vi "Plot 4 corners.vi"(8 "error in (no error)":errorcluster, 10 "4 corners":dbl[][][](array[numeric]), 11 "Refnum in":T1) -> (0 "error out":errorcluster, 3 "Refnum out":T1)   [LabVIEW 2011]
uses:
  <vilib>/vision/Image Controls.llb/IMAQ Image.ctl
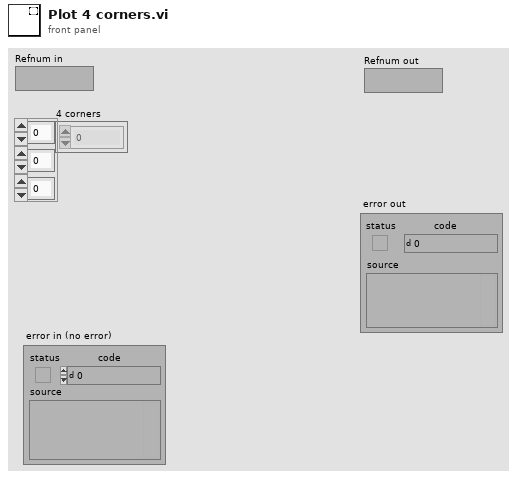
[diagram p1: front panel]
types:
  T1 = typedef "IMAQ Image.ctl" = refnum<image>
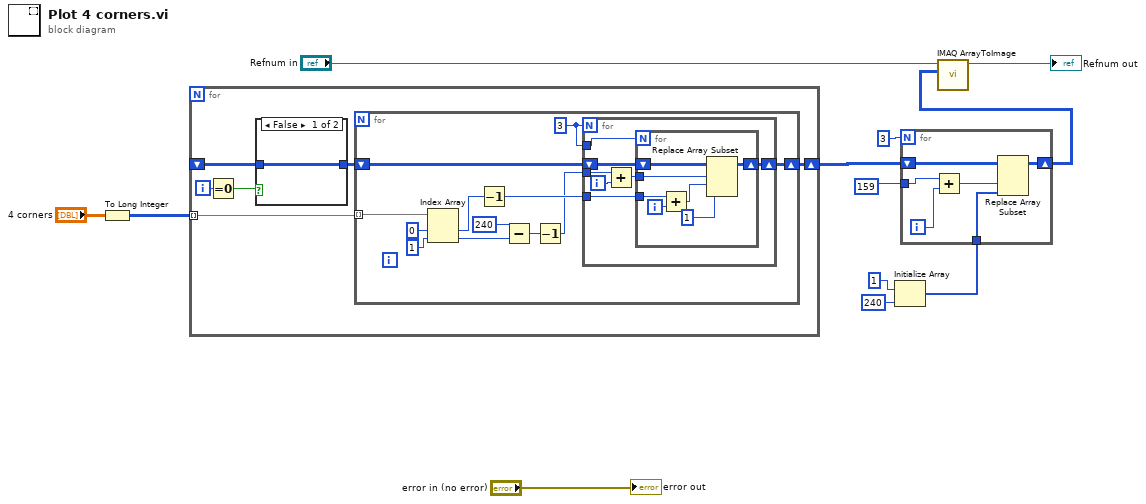
[diagram p0: block diagram]
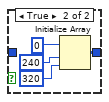
[diagram p2: hidden frame]
diagram:
  n1 = To Long Integer(number="4 corners") -> (32bit integer=w8:i32[][][])
  n2 = for {
    tunnel: w8 -> [w17] mode=indexing
    shift-right: [w16] -> w7
    shift-left: _ -> [w13]
    i -> [w15]
    n3 = Equal To 0?(x=w15) -> (x = 0?=w14:bool)
    n4 = case shown="False" w14 {
      tunnel: [w19 w20] -> w18
      tunnel: w13 -> [w19 _]
      frame False {
      }
      frame True {
        n5 = Initialize Array(u8 0, 240 ("dimension size"), 320 ("dimension size")) -> (w20:u8[][])
      }
    }
    n6 = for {
      tunnel: w17 -> [w35] mode=indexing
      shift-right: [w29] -> w16
      shift-left: w18 -> [w30]
      w24 = 3
      n7 = Index Array(array=w35, index #1=0 ("index"), index #2=1 ("index")) -> (element #1=w27:i32, element #2=w31:i32)
      n8 = Decrement(x=w27) -> (x-1=w26:i32)
      n9 = Subtract(x=240, y=w31) -> (x-y=w28:i32)
      n10 = Decrement(x=w28) -> (x-1=w25:i32)
      n11 = for {
        N: w24 -> [_]
        tunnel: w26 -> [w40]
        tunnel: w25 -> [w37]
        shift-right: [w41] -> w29
        shift-left: w30 -> [w42]
        tunnel: w24 -> [w39]
        i -> [w36]
        n12 = Add(x=w37, y=w36) -> (x+y=w38:i32)
        n13 = for {
          N: w39 -> [_]
          tunnel: w40 -> [w46]
          tunnel: w38 -> [w45]
          shift-right: [w48] -> w41
          shift-left: w42 -> [w49]
          i -> [w43]
          n14 = Add(x=w46, y=w43) -> (x+y=w44:i32)
          n15 = Replace Array Subset(array=w49, new element=u8 1 ("new element/subarray"), index (row)=w45, index (col)=w44) -> (w48:u8[][])
        }
      }
    }
  }
  n16 = Initialize Array(u8 1 ("new element/subarray"), 240 ("dimension size")) -> (w4:u8[])
  n17 = for {
    N: 3 -> [_]
    tunnel: w4 -> [w54]
    shift-right: [w53] -> w1
    shift-left: w7 -> [w55]
    tunnel: 159 ("disabled index (col)") -> [w51]
    i -> [w50]
    n18 = Add(x=w51, y=w50) -> (x+y=w52:i32)
    n19 = Replace Array Subset(array=w55, new element=w54, index (col)=w52) -> (w53:u8[][])  [unwired: 1 in]
  }
  n20 = call "IMAQ ArrayToImage"("Image Pixels (U8)"=w1, "Image"="Refnum in") -> ("Image Out"=→"Refnum out":T1)  [unwired: 8 in, 1 out]
  "error out" <- "error in (no error)"
